vi "FMDLDataWrite.vi"(1 "transpose? (no:F)":bool, 2 "append to file? (new file:F)":bool=TRUE, 3 "error in (no error)":errorcluster, 4 "1D data":dbl[](array[numeric]), 5 "2D data":dbl[][](array[numeric]), 6 "file path (dialog if empty)":path) -> (0 "error out":errorcluster)   [LabVIEW 2018]
uses:
  <vilib>/Utility/file.llb/Write Delimited Spreadsheet (DBL).vi
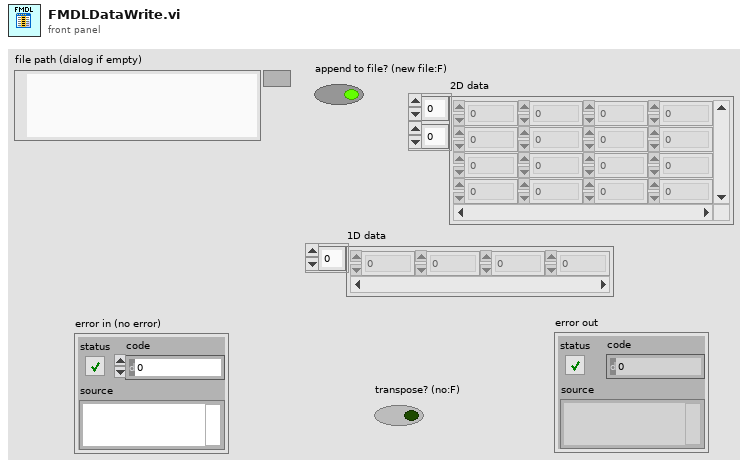
[diagram p1: front panel]
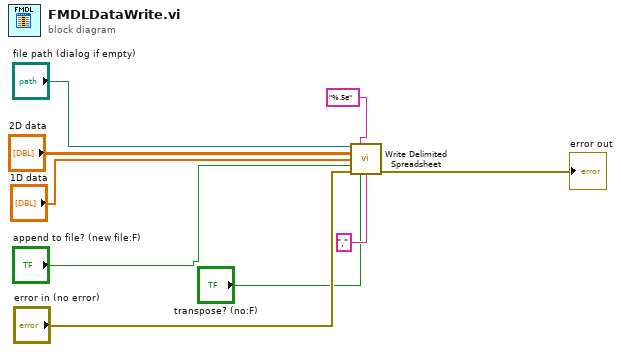
[diagram p0: block diagram]
diagram:
  n1 = call-poly <vilib>:"Write Delimited Spreadsheet.vi"("file path (dialog if empty)"="file path (dialog if empty)", "format (%.3f)"="%.5e", "2D data"="2D data", "1D data"="1D data", "append to file? (new file:F)"="append to file? (new file:F)", "error in (no error)"="error in (no error)", "transpose? (no:F)"="transpose? (no:F)", "delimiter (\\t)"=",") -> ("error out"=→"error out":errorcluster)  [unwired: 6 in, 1 out]
